vi "Create DataTable.vi"(8 "error in (no error)":errorcluster, 10 "String Data":string[][](array[string]), 11 "DataGridView in":refnum<class "DataGridView.lvclass">) -> (0 "error out":errorcluster, 3 "DataGridView out":refnum<class "DataGridView.lvclass">)   [LabVIEW 2014, in "DataGridView.lvclass"]
uses:
  DataGridView.lvclass
  DataGridView.lvclass/DataGridView.ctl
  System.Data
  GridColumn/GridColumn.lvclass/GridColumn.ctl
  GridColumn/Read datatype.vi
  GridColumn/Read Params.vi
  GridColumn/Read Name.vi
  GridColumn/GridColumn.lvclass
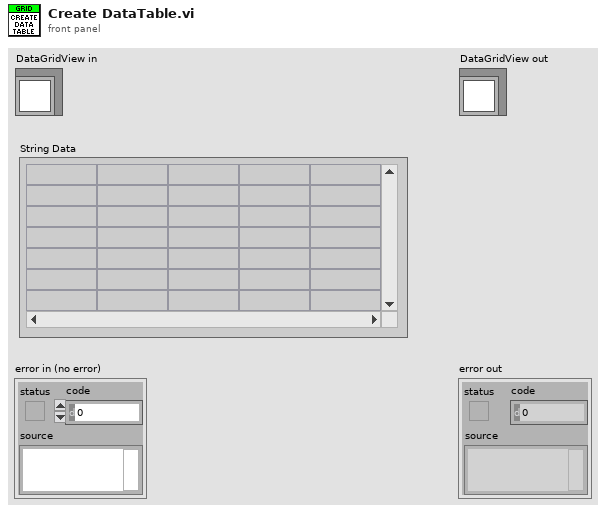
[diagram p1: front panel]
types:
  T1 = enum16{"string", "image", "check", "numeric", "timestamp", "button", "combo"}
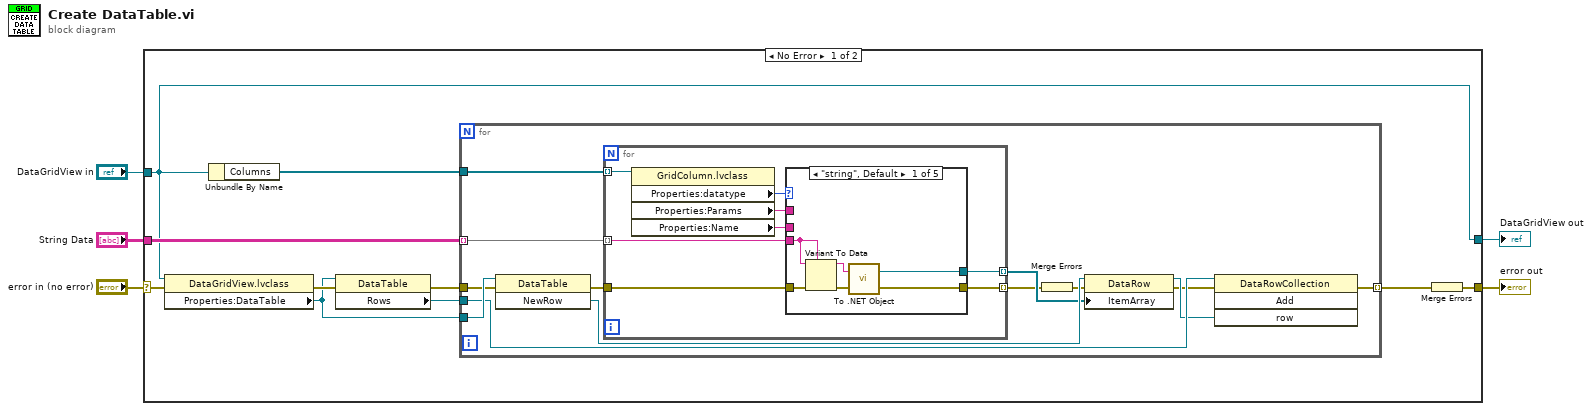
[diagram p0: block diagram]
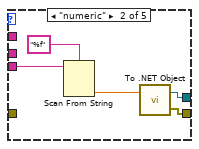
[diagram p2: hidden frame]
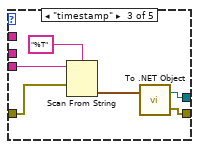
[diagram p3: hidden frame]
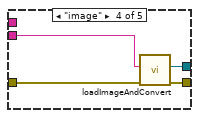
[diagram p4: hidden frame]
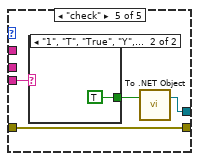
[diagram p5: hidden frame]
diagram:
  n1 = case shown="No Error" "error in (no error)" {
    selector: "error in (no error)" -> [w14 w64]
    tunnel: [w7 w64] -> w4
    tunnel: [w12 w63] -> w2
    tunnel: "DataGridView in" -> [w12 w63]
    tunnel: "String Data" -> [w13 _]
    frame No Error {
      n2 = property class="DataGridView.lvclass"(reference=w12, error in=w14) -> (error out=w9:errorcluster, "Properties:DataTable"=w6:refnum<k24>)  [unwired: 1 out]
      n3 = Unbundle By Name(w12) -> ("Columns"=w11:refnum<class "GridColumn.lvclass">[])
      n4 = property class="DataTable"(reference=w6, error in=w9) -> (error out=w8:errorcluster, "Rows"=w10:refnum<k24>)  [unwired: 1 out]
      n5 = for {
        tunnel: w10 -> [w27]
        tunnel: w6 -> [w28]
        tunnel: [w26] -> w15 mode=indexing
        tunnel: w13 -> [w25] mode=indexing
        tunnel: w8 -> [w17]
        tunnel: w11 -> [w16]
        n6 = invoke class="DataTable" method="NewRow"(reference=w28, error in=w17) -> (error out=w24:errorcluster, "NewRow"=w23:refnum<k24>)  [unwired: 1 in, 1 out]
        n7 = for {
          tunnel: w25 -> [w36] mode=indexing
          tunnel: [w35] -> w21 mode=indexing
          tunnel: w24 -> [w34]
          tunnel: [w33] -> w20 mode=indexing
          tunnel: w16 -> [w32] mode=indexing
          n8 = property class="GridColumn.lvclass"(reference=w32) -> ("Properties:datatype"=w31:T1, "Properties:Params"=w30:string, "Properties:Name"=w29:string)  [unwired: 1 in, 2 out]
          n9 = case shown="\"string\", Default" w31 {
            tunnel: w36 -> [w38 w45 w51 w57 w59]
            tunnel: [w37 w46 w52 w56 w60] -> w35
            tunnel: w34 -> [w41 _ w49 w55 w61]
            tunnel: [w39 w47 w53 w54 w61] -> w33
            tunnel: w30 -> [_ _ _ _ _]
            tunnel: w29 -> [_ _ _ _ _]
            frame "string", Default {
              n10 = Variant To Data(error in=w41, type=w38, Variant=w38) -> (data=w42:string, error out=w40:errorcluster)
              n11 = call <vilib>:"To .NET Object.vi"("error in (no error)"=w40, "anything"=w42) -> ("error out"=w39:errorcluster, ".NET object"=w37:refnum<k24>)
            }
            frame "numeric" {
              n12 = Scan From String(format string="%f", input string=w45) -> (output 1=w43:dbl)  [unwired: 3 in, 3 out]
              n13 = call <vilib>:"To .NET Object.vi"("anything"=w43) -> ("error out"=w47:errorcluster, ".NET object"=w46:refnum<k24>)  [unwired: 1 in]
            }
            frame "timestamp" {
              n14 = Scan From String(format string="%T", input string=w51, error in=w49) -> (output 1=w48:timestamp)  [unwired: 2 in, 3 out]
              n15 = call <vilib>:"To .NET Object.vi"("anything"=w48) -> ("error out"=w53:errorcluster, ".NET object"=w52:refnum<k24>)  [unwired: 1 in]
            }
            frame "image" {
              n16 = call "loadImageAndConvert.vi"("error in (no error)"=w55, "name or relative path"=w57) -> ("error out"=w54:errorcluster, ".NET object"=w56:refnum<k24>)  [unwired: 8 in]
            }
            frame "check" {
              n17 = case shown="\"1\", \"T\", \"True\", \"Y\", \"Yes\"" w59 {
                tunnel: [_ TRUE] -> w58
                frame Default {
                }
                frame "1", "T", "True", "Y", "Yes" {
                }
              }
              n18 = call <vilib>:"To .NET Object.vi"("anything"=w58) -> (".NET object"=w60:refnum<k24>)  [unwired: 1 in, 1 out]
            }
          }
        }
        n19 = Merge Errors(w20) -> (w19:errorcluster)
        n20 = property class="DataRow"(reference=w23, error in=w19, "ItemArray"=w21) -> (reference out=w22:refnum<k24>, error out=w18:errorcluster)
        n21 = invoke class="DataRowCollection" method="Add"(reference=w27, error in=w18, "row"=w22) -> (error out=w26:errorcluster)  [unwired: 1 in, 3 out]
      }
      n22 = Merge Errors(w15) -> (w7:errorcluster)
    }
    frame Error {
    }
  }
  "error out" <- w4
  "DataGridView out" <- w2
